vi "set_next.vi"(8 "error in (no error)":errorcluster, 10 "next":refnum<class "Iterator.lvclass">, 11 "DoublyNodeRef in":refnum<class "Iterator.lvclass">) -> (0 "error out":errorcluster, 3 "DoublyNodeRef out":refnum<class "Iterator.lvclass">)   [LabVIEW 2021, in "Iterator.lvclass"]
uses:
  Iterator.lvclass
  Iterator.lvclass/Iterator.ctl
  IDoublyNode/IDoublyNode.lvclass
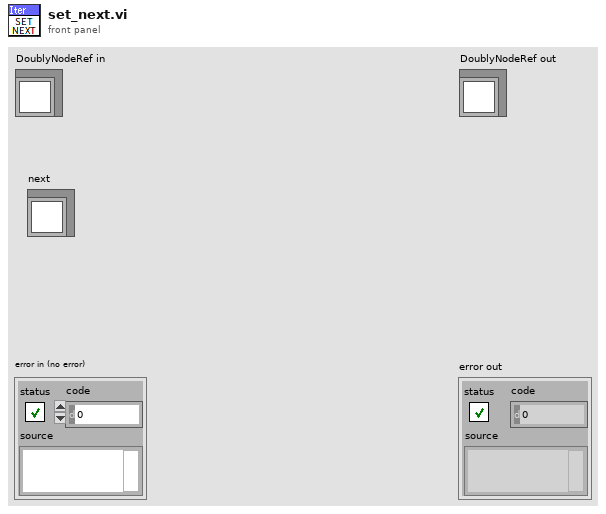
[diagram p1: front panel]
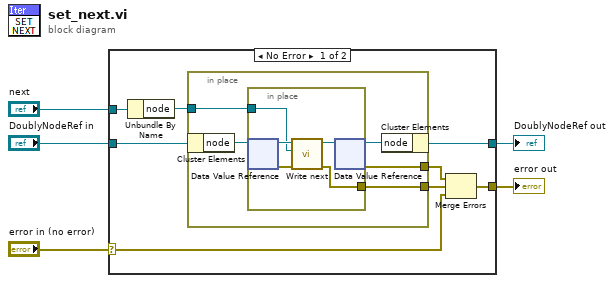
[diagram p0: block diagram]
diagram:
  n1 = case shown="No Error" "error in (no error)" {
    selector: "error in (no error)" -> [w7 w25]
    tunnel: [w6 w25] -> w4
    tunnel: [w10 w24] -> w2
    tunnel: "DoublyNodeRef in" -> [w13 w24]
    tunnel: "next" -> [w12 _]
    frame No Error {
      n2 = Unbundle By Name(w12) -> ("node"=w11:refnum<data-value>)
      n3 = in-place {
        in-place-border: [w16] -> w9
        in-place-border: w11 -> [w15]
        in-place-border: [w14] -> w8
        n4 = in-place-cluster #1(w13) -> ("node"=w18:refnum<data-value>)
        n5 = in-place {
          in-place-border: w15 -> [w20]
          in-place-border: [w19] -> w14
          n6 = in-place-dvr #2(w18) -> (w23:refnum<class "IDoublyNode.lvclass">, w21:errorcluster)
          n7 = call-dynamic "Write next.vi"("error in (no error)"=w21, "next"=w20, "NodeType in"=w23) -> ("error out"=w19:errorcluster, "NodeType out"=w22:refnum<class "IDoublyNode.lvclass">)  [unwired: 7 in]
          n8 = in-place-dvr #2(w22) -> (w17:refnum<data-value>, w16:errorcluster)
        }
        n9 = in-place-cluster #1("node"=w17) -> (w10:refnum<class "Iterator.lvclass">)
      }
      n10 = Merge Errors(w9, w8, w7) -> (w6:errorcluster)
    }
    frame Error {
    }
  }
  "error out" <- w4
  "DoublyNodeRef out" <- w2
